vi "Hydrosonic_Conrol.vi"(2 "In range %":dbl format="%.2f", 3 "Input Mode":enum16{"Desired Frequency", "Transducer value"}(ring), 4 "Actual Sampling rate (Hz)":dbl=1000.0 format="%.2f", 5 "Desired Value":dbl format="%.2f") -> (0 "Error Info":string, 1 "Set output":dbl format="%.2f")   [LabVIEW 2020]
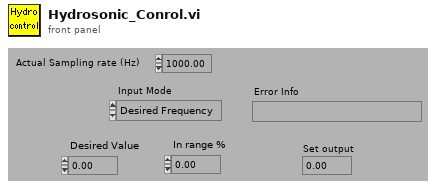
[diagram p1: front panel]
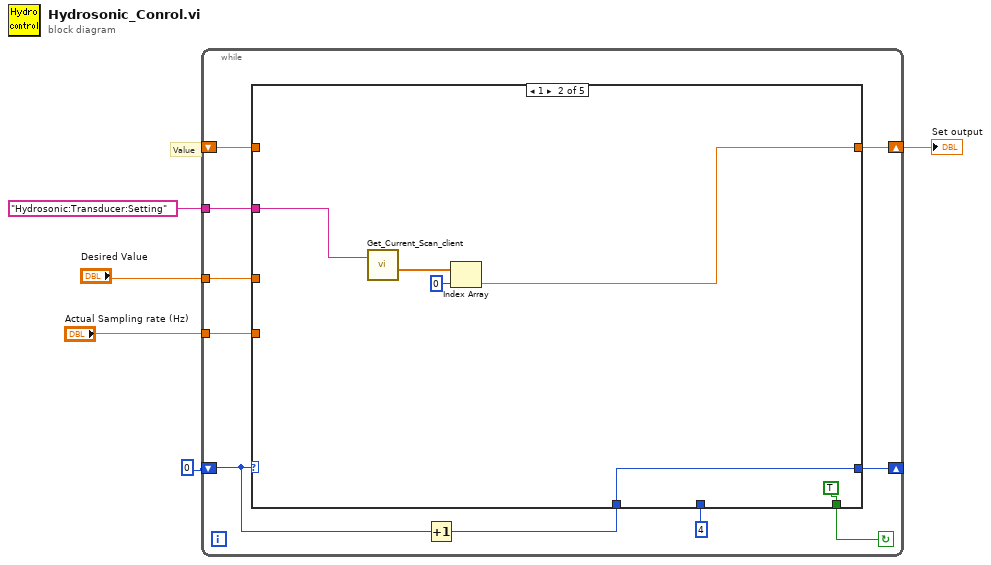
[diagram p0: block diagram]
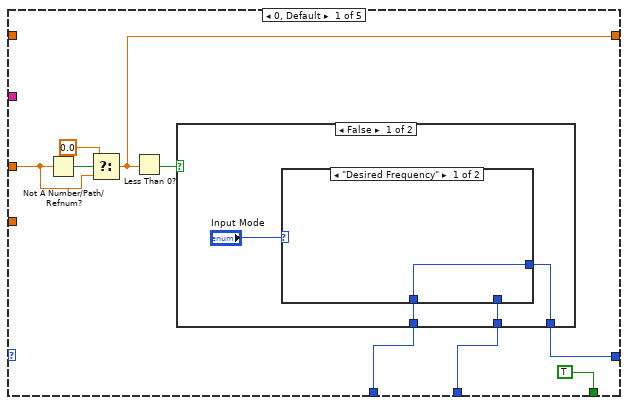
[diagram p2: hidden frame]
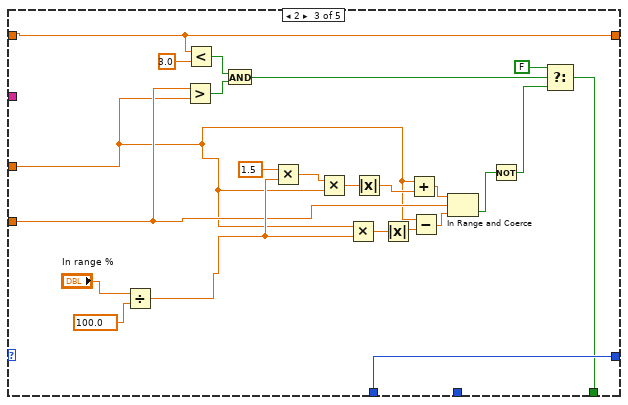
[diagram p5: hidden frame]
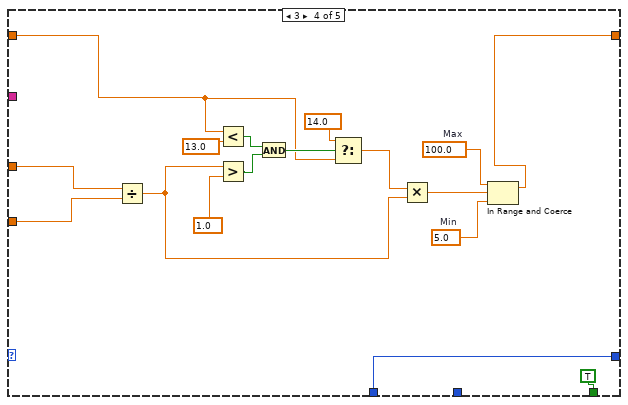
[diagram p6: hidden frame]
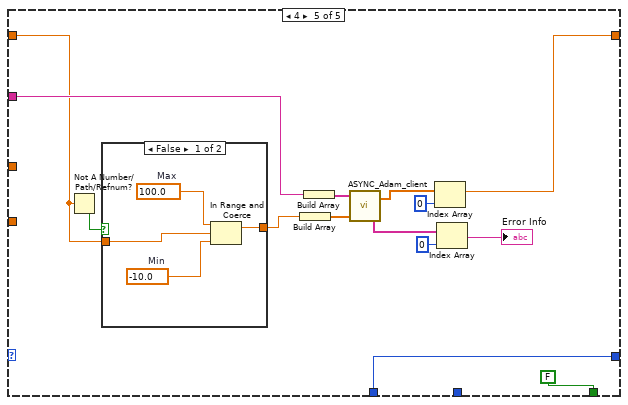
[diagram p7: hidden frame]
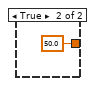
[diagram p8: hidden frame]
diagram:
  # "Value"
  n1 = while {
    tunnel: "Actual Sampling rate (Hz)" -> [w8]
    tunnel: "Hydrosonic:Transducer:Setting" -> [w10]
    shift-left: _ -> [w7]
    shift-right: [w9] -> w1
    tunnel: "Desired Value" -> [w15]
    shift-left: 0 -> [w14]
    shift-right: [w13] -> _
    stop <- w11 continue-if-true
    n2 = Increment(x=w14) -> (x+1=w12:i32)
    n3 = case shown="1" w14 {
      tunnel: w15 -> [w19 _ w46 w75 _]
      tunnel: [w24 w34 w60 w77 w90] -> w13
      tunnel: w12 -> [w23 w34 w60 w77 w90]
      tunnel: [TRUE TRUE w38 TRUE FALSE] -> w11
      tunnel: w10 -> [_ w32 _ _ w84]
      tunnel: [w16 w35 w45 w61 w81] -> w9
      tunnel: w8 -> [_ _ w47 w74 _]
      tunnel: w7 -> [_ _ w45 w67 w79]
      tunnel: 4 -> [w21 _ _ _ _]
      frame 0, Default {
        n4 = Not A Number/Path/Refnum?(number/path/refnum=w19) -> (NaN/Path/Refnum?=w20:bool)
        n5 = Select(t=0.0, s=w20, f=w19) -> (s? t:f=w16:dbl)
        n6 = Less Than 0?(x=w16) -> (x < 0?=w17:bool)
        n7 = case shown="False" w17 {
          tunnel: [w27 w31] -> w24
          tunnel: w23 -> [w26 _]
          tunnel: w21 -> [w25 w31]
          frame False {
            n8 = case shown="\"Desired Frequency\"" "Input Mode" {
              tunnel: [w29 w30] -> w27
              tunnel: w26 -> [w29 _]
              tunnel: w25 -> [_ w30]
              frame "Desired Frequency" {
              }
              frame "Transducer value" {
              }
            }
          }
          frame True {
          }
        }
      }
      frame 1 {
        n9 = call "Get_Current_Scan_client.vi"("singleChannel"=w32) -> ("Numerical Values"=w37:dbl[])  [unwired: 2 in, 2 out]
        n10 = Index Array(array=w37, index=0 ("Index")) -> (element=w35:dbl)
      }
      frame 2 {
        n11 = Divide(x="In range %", y=100.0) -> (x/y=w52:dbl)
        n12 = Greater?(x=w47, y=w46) -> (0:w43:bool)
        n13 = Less?(x=w45, y=3.0) -> (x < y?=w42:bool)
        n14 = And(x=w42, y=w43) -> (x .and. y?=w40:bool)
        n15 = Multiply(x=1.5, y=w52) -> (x*y=w50:dbl)
        n16 = Multiply(x=w50, y=w46) -> (x*y=w51:dbl)
        n17 = Multiply(x=w46, y=w52) -> (x*y=w57:dbl)
        n18 = Absolute Value(x=w51) -> (abs(x)=w49:dbl)
        n19 = Absolute Value(x=w57) -> (abs(x)=w54:dbl)
        n20 = Add(x=w46, y=w49) -> (x+y=w59:dbl)
        n21 = Subtract(x=w46, y=w54) -> (x-y=w58:dbl)
        n22 = In Range and Coerce(upper limit=w59, x=w47, lower limit=w58) -> (In Range?=w48:bool)  [unwired: 1 out]
        n23 = Not(x=w48) -> (.not. x?=w41:bool)
        n24 = Select(t=FALSE, s=w40, f=w41) -> (s? t:f=w38:bool)
      }
      frame 3 {
        w63 = 100.0  # Max
        w64 = 5.0  # Min
        n25 = Divide(x=w75, y=w74) -> (x/y=w65:dbl)
        n26 = Less?(x=w67, y=13.0) -> (x < y?=w70:bool)
        n27 = Greater?(x=w65, y=1.0) -> (0:w71:bool)
        n28 = And(x=w70, y=w71) -> (x .and. y?=w69:bool)
        n29 = Select(t=14.0, s=w69, f=w67) -> (s? t:f=w66:dbl)
        n30 = Multiply(x=w66, y=w65) -> (x*y=w62:dbl)
        n31 = In Range and Coerce(upper limit=w63, x=w62, lower limit=w64) -> (coerced(x)=w61:dbl)  [unwired: 1 out]
      }
      frame 4 {
        n32 = Not A Number/Path/Refnum?(number/path/refnum=w79) -> (NaN/Path/Refnum?=w80:bool)
        n33 = case shown="False" w80 {
          tunnel: w79 -> [w93 _]
          tunnel: [w92 50.0 ("Max")] -> w82
          frame False {
            w94 = 100.0  # Max
            w95 = -10.0  # Min
            n34 = In Range and Coerce(upper limit=w94, x=w93, lower limit=w95) -> (coerced(x)=w92:dbl)  [unwired: 1 out]
          }
          frame True {
          }
        }
        n35 = Build Array(w82) -> (w87:dbl[])
        n36 = Build Array(w84) -> (w78:string[])
        n37 = call "ASYNC_Adam_client.vi"("Values"=w87, "Channel Names"=w78) -> ("Scan Comments"=w85:string[], "Calibrated Units"=w86:dbl[])  [unwired: 1 in]
        n38 = Index Array(array=w86, index=0 ("Index")) -> (element=w81:dbl)
        n39 = Index Array(array=w85, index=0 ("Index")) -> (element=→"Error Info":string)
      }
    }
  }
  "Set output" <- w1
